vi "Analytical Inverse Kinematics (5R Type 1).vi"(8 "error in (no error)":errorcluster, 10 "end effector transform":T1, 11 "5R type 1 serial arm in":refnum<class "NI_Robotics_5R Type 1 Serial Arm Class.lvclass">) -> (0 "error out":errorcluster, 1 "reachable":bool, 2 "joint positions":T1, 3 "5R type 1 serial arm out":refnum<class "NI_Robotics_5R Type 1 Serial Arm Class.lvclass">)   [LabVIEW 2017, in "NI_Robotics_5R Type 1 Serial Arm Class.lvclass"]
doc: "Returns the joint angles of a 6R, 5R, or SCARA arm given the posture of the end effector relative to the arm base. Wire data to the <B>X</B><B>_serial arm in</B> input, where <B>X</B> is the arm type, to determine the polymorphic instance to use or manually select the instance."
uses:
  <vilib>/robotics/Kinematics/Analytical/5R/Type 1/NI_Robotics_5R Type 1 Serial Arm Class.lvclass
  c:/Program Files (x86)/National Instruments/LabVIEW 2017/vi.lib/robotics/Kinematics/Robot/NI_Robotics_Serial Robot Arm.lvclass
  <vilib>/Analysis/Matrix/Datatypes/RealMatrix.ctl
  <vilib>/robotics/Kinematics/Analytical/5R/Type 1/NI_Robotics_5R Type 1 Serial Arm Class.lvclass/NI_Robotics_5R Type 1 Serial Arm Class.ctl
  <vilib>/Analysis/baseanly.llb/Real A x B.vi
  <vilib>/Analysis/baseanly.llb/A x Vector.vi
  <vilib>/Analysis/coordinate.llb/Wrap Angle (array).vi
  <vilib>/robotics/Kinematics/RotateX.vi
  <vilib>/robotics/Kinematics/RotateY.vi
  <vilib>/robotics/Kinematics/RotateZ.vi
  <vilib>/Analysis/baseanly.llb/Real Inverse Matrix.vi
  <vilib>/robotics/Kinematics/Robot/NI_Robotics_Serial Robot Arm.lvclass
  <vilib>/Analysis/NI_AALBase.lvlib
  <vilib>/robotics/Kinematics/NI_Kinematics.lvlib
  <vilib>/Analysis/NI_AAL_Angle.lvlib
  <vilib>/Analysis/Matrix/NI_Matrix.lvlib
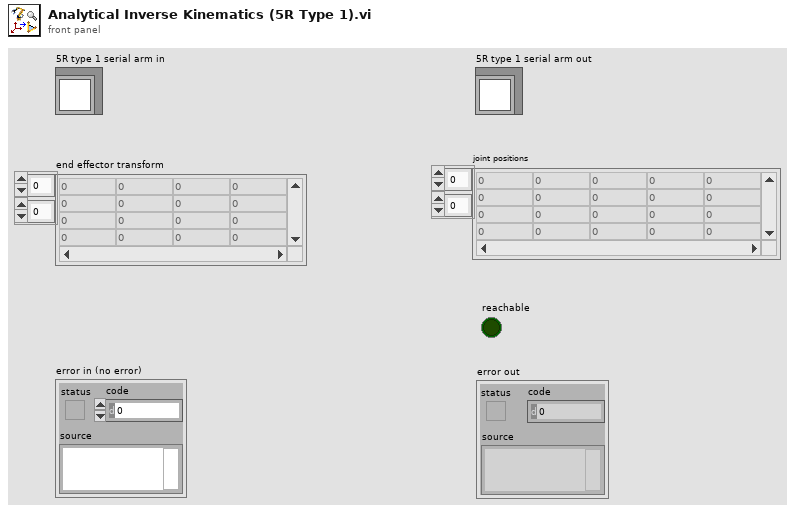
[diagram p1: front panel]
types:
  T1 = typedef "NI_Matrix.lvlib/RealMatrix.ctl" = dbl[][]
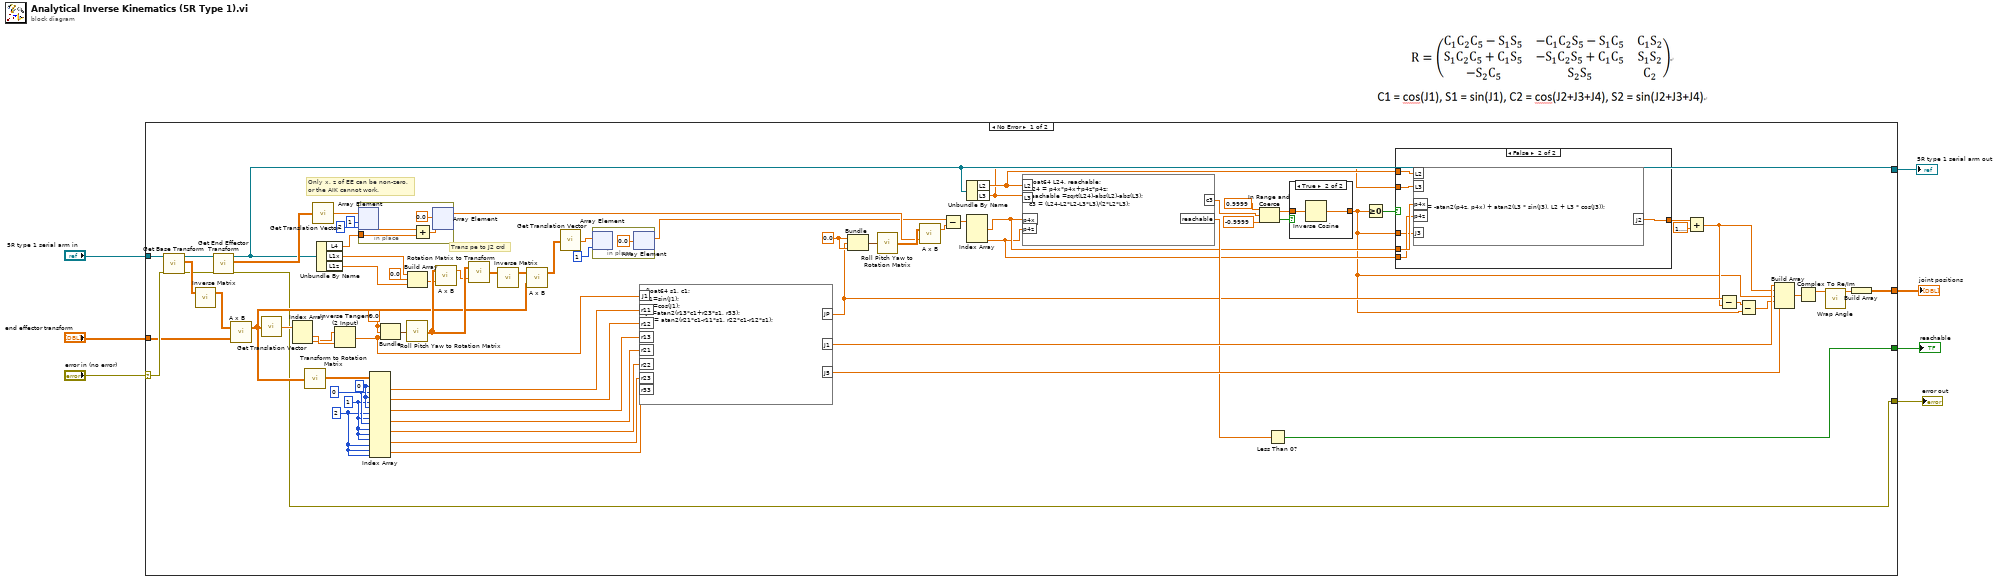
[diagram p0: block diagram]
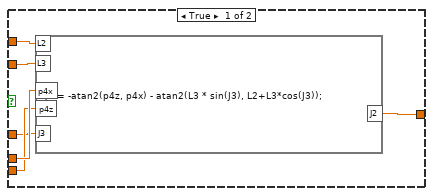
[diagram p2: hidden frame]
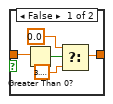
[diagram p3: hidden frame]
diagram:
  n1 = case shown="No Error" "error in (no error)" {
    selector: "error in (no error)" -> [w79 w108]
    tunnel: [w29 w108] -> w6
    tunnel: [w50 w109] -> w4
    tunnel: "5R type 1 serial arm in" -> [w80 w109]
    tunnel: "end effector transform" -> [w77 _]
    tunnel: [w27 _] -> w2
    tunnel: [w46 _] -> w1
    frame No Error {
      w34 = 2 ("disabled index (col)")
      w38 = 1 ("disabled index (col)")
      w39 = 0 ("disabled index (col)")
      w43 = 0 ("index (row)")
      w59 = 0.0
      w73 = 0.0
      # "Trans pe to J2 crd"
      # "Only x, z of EE can be non-zero, \nor the AIK cannot work."
      n2 = call <vilib>:"Get Base Transform.vi"("error in (no error)"=w79, "serial arm in"=w80) -> ("error out"=w81:errorcluster, "base transform"=w82:T1, "serial arm out"=w83:refnum<class "NI_Robotics_5R Type 1 Serial Arm Class.lvclass">)  [unwired: 7 in]
      n3 = call-poly <vilib>:"Inverse Matrix.vi"("Input Matrix"=w82) -> ("Inverse Matrix"=w78:T1)  [unwired: 1 in, 1 out]
      n4 = call <vilib>:"Get End Effector Transform.vi"("error in (no error)"=w81, "serial arm in"=w83) -> ("error out"=w29:errorcluster, "end effector transform"=w76:T1, "serial arm out"=w50:refnum<class "NI_Robotics_5R Type 1 Serial Arm Class.lvclass">)  [unwired: 7 in]
      n5 = call-poly <vilib>:"A x B.vi"("B"=w77, "A"=w78) -> ("A x B"=w60:T1)  [unwired: 1 out]
      n6 = call <vilib>:"Get Translation Vector.vi"("transform"=w60) -> ("translation vector"=w75:dbl[])
      n7 = Index Array(array=w75) -> (element #1=w65:dbl, element #2=w45:dbl)  [unwired: 2 in]
      n8 = call <vilib>:"Transform to Rotation Matrix.vi"("transform"=w60) -> ("rotation matrix"=w44:T1)
      n9 = call <vilib>:"Get Translation Vector.vi"("transform"=w76) -> ("translation vector"=w62:dbl[])
      n10 = Unbundle By Name(w50) -> ("L4"=w8:dbl, "L1x"=w64:dbl, "L1z"=w63:dbl)
      n11 = Inverse Tangent (2 Input)(1:w65, 2:w45) -> (0:w32:dbl)
      n12 = in-place {
        in-place-border: w8 -> [w104]
        n13 = in-place-array #1(w62, 1, 2) -> (w106:dbl)  [unwired: 1 out]
        n14 = Add(x=w106, y=w104) -> (x+y=w105:dbl)
        n15 = in-place-array #1(0.0 ("element"), w105) -> (w56:dbl[])  [unwired: 2 out]
      }
      n16 = Index Array(array=w44, index (row) #1=w43, index (col) #1=w39, index (row) #2=w43, index (col) #2=w38, index (row) #3=w43, index (col) #3=w34, index (row) #4=w38, index (col) #4=w39, index (row) #5=w38, index (col) #5=w38, index (row) #6=w38, index (col) #6=w34, index (row) #7=w34, index (col) #7=w34) -> (element #1=w42:dbl, element #2=w41:dbl, element #3=w40:dbl, element #4=w37:dbl, element #5=w36:dbl, element #6=w35:dbl, element #7=w33:dbl)
      n17 = Bundle(w73, w73, w32) -> (w72:cluster{dbl, dbl, dbl})  [unwired: 1 in]
      n18 = call <vilib>:"Roll Pitch Yaw to Rotation Matrix.vi"("angles"=w72) -> ("rotation matrix"=w68:T1)
      n19 = Build Array(w64, 0.0 ("element"), w63) -> (w67:dbl[])
      n20 = call-poly <vilib>:"A x B.vi"("Vector"=w67, "A"=w68) -> ("A x Vector"=w66:dbl[])  [unwired: 1 out]
      n21 = call <vilib>:"Rotation Matrix to Transform.vi"("translation vector"=w66, "rotation matrix"=w68) -> ("transform"=w71:T1)
      n22 = call-poly <vilib>:"Inverse Matrix.vi"("Input Matrix"=w71) -> ("Inverse Matrix"=w69:T1)  [unwired: 1 in, 1 out]
      n23 = call-poly <vilib>:"A x B.vi"("B"=w60, "A"=w69) -> ("A x B"=w70:T1)  [unwired: 1 out]
      n24 = call <vilib>:"Get Translation Vector.vi"("transform"=w70) -> ("translation vector"=w54:dbl[])
      n25 = in-place {
        n26 = in-place-array #2(w54, 1) -> ()  [unwired: 1 out]
        n27 = in-place-array #2(0.0 ("element")) -> (w52:dbl[])  [unwired: 1 out]
      }
      n28 = formula code="float64 s1, c1;\ns1=sin(J1);\nc1=cos(J1);\nJP=atan2(r13*c1+r23*s1, r33);\nJ5 = atan2(r21*c1-r11*s1, r22*c1-r12*s1);"("J1"=w32, "r11"=w42, "r12"=w41, "r13"=w40, "r21"=w37, "r22"=w36, "r23"=w35, "r33"=w33) -> ("JP"=w15:dbl, "J1"=w30:dbl, "J5"=w31:dbl)
      n29 = Bundle(w59, "JP"=w15, w59) -> (w58:cluster{dbl, "JP":dbl, dbl})  [unwired: 1 in]
      n30 = call <vilib>:"Roll Pitch Yaw to Rotation Matrix.vi"("angles"=w58) -> ("rotation matrix"=w57:T1)
      n31 = call-poly <vilib>:"A x B.vi"("Vector"=w56, "A"=w57) -> ("A x Vector"=w55:dbl[])  [unwired: 1 out]
      n32 = Subtract(x=w52, y=w55) -> (x-y=w51:dbl[])
      n33 = Unbundle By Name(w50) -> ("L2"=w21:dbl, "L3"=w20:dbl)
      n34 = Index Array(array=w51) -> (element #1=w19:dbl, element #3=w18:dbl)  [unwired: 3 in, 1 out]
      n35 = formula code="float64 L24, reachable;\nL24 = p4x*p4x+p4z*p4z;\nreachable =sqrt(L24)-abs(L2)-abs(L3);\nc3 = (L24-L2*L2-L3*L3)/(2*L2*L3);"("p4x"=w19, "p4z"=w18, "L2"=w21, "L3"=w20) -> ("c3"=w10:dbl, "reachable"=w28:dbl)
      n36 = In Range and Coerce(upper limit=0.9999, x=w10, lower limit=-0.9999) -> (coerced(x)=w23:dbl, In Range?=w24:bool)
      n37 = Less Than 0?(x=w28) -> (x < 0?=w27:bool)
      n38 = case shown="True" w24 {
        tunnel: w23 -> [w100 w102]
        tunnel: [w96 w101] -> w12
        frame False {
          n39 = Greater Than 0?(x=w100) -> (x > 0?=w99:bool)
          n40 = Select(t=0.0, s=w99, f=3.141592653589793) -> (s? t:f=w96:dbl)
        }
        frame True {
          n41 = Inverse Cosine(1:w102) -> (0:w101:dbl)
        }
      }
      n42 = Greater Or Equal To 0?(x=w12) -> (x >= 0?=w22:bool)
      n43 = case shown="False" w22 {
        tunnel: w21 -> [w89 w95]
        tunnel: w20 -> [w88 w94]
        tunnel: w19 -> [w87 w93]
        tunnel: w18 -> [w86 w92]
        tunnel: w12 -> [w85 w91]
        tunnel: [w84 w90] -> w17
        frame True {
          n44 = formula code="J2 = -atan2(p4z, p4x) - atan2(L3 * sin(J3), L2+L3*cos(J3));"("p4x"=w87, "p4z"=w86, "J3"=w85, "L2"=w89, "L3"=w88) -> ("J2"=w84:dbl)
        }
        frame False {
          n45 = formula code="J2 = -atan2(p4z, p4x) + atan2(L3 * sin(J3), L2 + L3 * cos(J3));"("p4x"=w93, "p4z"=w92, "J3"=w91, "L2"=w95, "L3"=w94) -> ("J2"=w90:dbl)
        }
      }
      n46 = Add(x=w17, y=1.5707963267948966) -> (x+y=w14:dbl)
      n47 = Subtract(x=w15, y=w14) -> (x-y=w13:dbl)
      n48 = Subtract(x=w13, y=w12) -> (x-y=w11:dbl)
      n49 = Build Array(w30, w14, w12, w11, w31) -> (w49:dbl[])
      n50 = Complex To Re/Im(x + iy=w49) -> (x=w48:dbl[])  [unwired: 1 out]
      n51 = call-poly <vilib>:"Wrap Angle.vi"("Angle In"=w48) -> ("Angle Out"=w47:dbl[])  [unwired: 9 in, 1 out]
      n52 = Build Array(w47) -> (w46:dbl[][])
    }
    frame Error {
    }
  }
  "error out" <- w6
  "5R type 1 serial arm out" <- w4
  "joint positions" <- w1
  "reachable" <- w2
